vi "CRC.vi"(1 "StrIn":string) -> (0 "StrOut":string)   [LabVIEW 2013]
panel:
  out "数组":u32[](array[numeric])
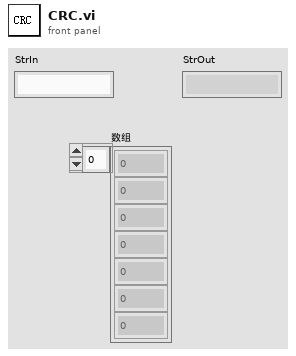
[diagram p1: front panel]
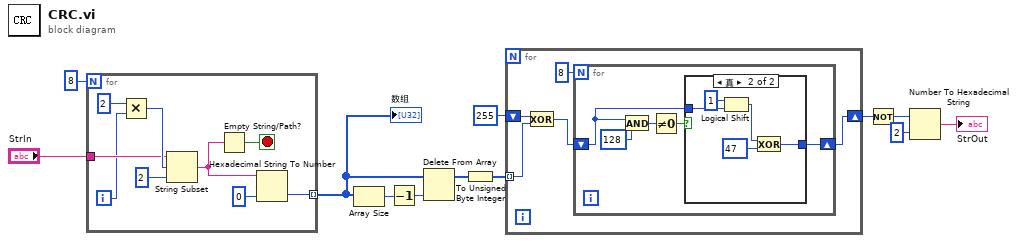
[diagram p0: block diagram]
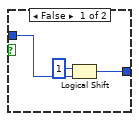
[diagram p2: hidden frame]
diagram:
  n1 = for {
    N: 8 -> [_]
    tunnel: "StrIn" -> [w18]
    tunnel: [w15] -> w6 mode=indexing
    i -> [w16]
    stop <- w17 stop-if-true
    n2 = Multiply(x=2, y=w16) -> (x*y=w20:i32)
    n3 = String Subset(string=w18, offset (0)=w20, length (rest)=2 ("length (rest)")) -> (substring=w13:string)
    n4 = Empty String/Path?(string/path=w13) -> (empty?=w17:bool)
    n5 = Hexadecimal String To Number(string=w13, default (0uL)=u32 0 ("默认值 1")) -> (number=w15:u32)  [unwired: 1 in, 1 out]
  }
  "数组" <- w6
  n6 = Array Size(array=w6) -> (size(s)=w5:i32)
  n7 = Decrement(x=w5) -> (x-1=w4:i32)
  n8 = Delete From Array(array=w6, index=w4) -> (array with subset deleted=w3:u32[])  [unwired: 1 in, 1 out]
  n9 = To Unsigned Byte Integer(number=w3) -> (unsigned 8bit integer=w2:u8[])
  n10 = for {
    shift-right: [w22] -> w9
    shift-left: u8 255 -> [w26]
    tunnel: w2 -> [w25] mode=indexing
    n11 = Exclusive Or(1:w25, 2:w26) -> (0:w23:u8)
    n12 = for {
      N: 8 -> [_]
      shift-right: [w28] -> w22
      shift-left: w23 -> [w27]
      n13 = And(x=w27, y=u8 128) -> (x .and. y?=w30:u8)
      n14 = Not Equal To 0?(x=w30) -> (x != 0?=w29:bool)
      n15 = case shown="真" w29 {
        tunnel: w27 -> [w32 w39]
        tunnel: [w34 w35] -> w28
        frame False {
          n16 = Logical Shift(y=1, x=w32) -> (x << y=w34:u8)
        }
        frame True {
          n17 = Logical Shift(y=1, x=w39) -> (x << y=w37:u8)
          n18 = Exclusive Or(1:u8 47, 2:w37) -> (0:w35:u8)
        }
      }
    }
  }
  n19 = Not(x=w9) -> (.not. x?=w1:u8)
  n20 = Number To Hexadecimal String(1:i16 2 ("宽度(-)"), 2:w1) -> (0:→"StrOut":string)
